vi "Autotest_Instr.vi"(8 "error in (no error)":errorcluster caption="entrée d'erreur (pas d'erreur)", 11 "Class Instrument Patterm_Matching en entrée":refnum<class "Class Instrument Patterm_Matching.lvclass">) -> (0 "error out":errorcluster caption="sortie d'erreur", 3 "Class Instrument Patterm_Matching en sortie":refnum<class "Class Instrument Patterm_Matching.lvclass">)   [LabVIEW 2020, in "Library Instrument & Equipement.lvlib" / "Library Instruments.lvlib" / "Class Instrument Patterm_Matching.lvclass"]
uses:
  Class Instrument Patterm_Matching.lvclass
  C:/Users/ngarcin/OneDrive - Altyor/Standard TB/Class/Instrument/Instrument (Default)/Class Instrument (Default).lvclass
  Class Instrument Patterm_Matching.lvclass/Class Instrument Patterm_Matching.ctl
  Instrument (Default)/Class Instrument (Default).lvclass
  Camera/Class Camera Pattern Matching (Default)/Class Pattern Matching (Default).lvclass
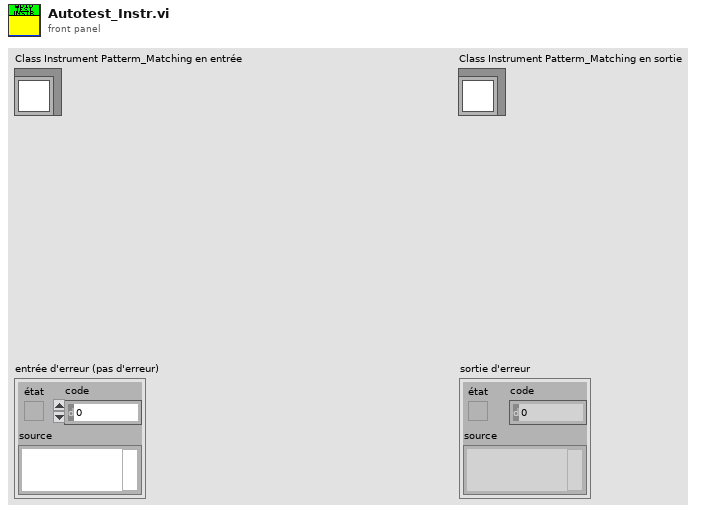
[diagram p1: front panel]
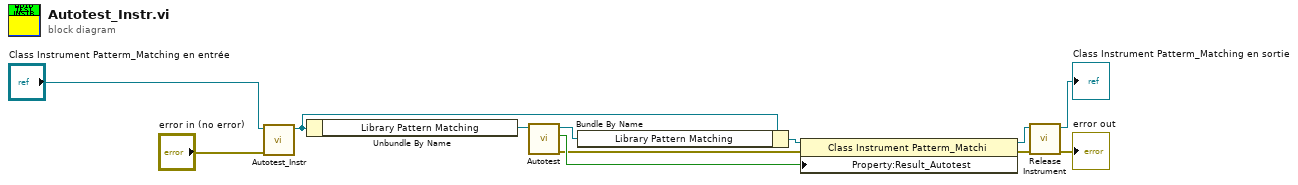
[diagram p0: block diagram]
diagram:
  n1 = call-parent "Autotest_Instr.vi"("error in (no error)"="error in (no error)", "Class Instrument (Default) en entrée"="Class Instrument Patterm_Matching en entrée") -> ("Class Instrument (Default) en sortie"=w8:refnum<class "Class Instrument Patterm_Matching.lvclass">)  [unwired: 8 in, 1 out]
  n2 = Unbundle By Name(w8) -> ("Library Pattern Matching"=w10:refnum<class "Class Pattern Matching (Default).lvclass">)
  n3 = call-dynamic "Autotest.vi"("Class Pattern Matching (Default) en entrée"=w10) -> ("error out"=w5:errorcluster, "Autotest"=w7:bool, "Class Pattern Matching (Default) en sortie"=w9:refnum<class "Class Pattern Matching (Default).lvclass">)  [unwired: 8 in]
  n4 = Bundle By Name(cluster=w8, "Library Pattern Matching"=w9) -> (w6:refnum<class "Class Instrument Patterm_Matching.lvclass">)
  n5 = property class="Class Instrument Patterm_Matchi"(reference=w6, error in=w5, "Property:Result_Autotest"=w7) -> (reference out=w3:refnum<class "Class Instrument Patterm_Matching.lvclass">, error out=w4:errorcluster)
  n6 = call-dynamic "Release Instrument.vi"("error in (no error)"=w4, "Class Instrument (Default) en entrée"=w3) -> ("error out"=→"error out":errorcluster, "Class Instrument (Default) en sortie"=→"Class Instrument Patterm_Matching en sortie":refnum<class "Class Instrument Patterm_Matching.lvclass">)  [unwired: 8 in]
